vi "Repeat_Meas_if_Unsteady.vi"() -> (5 "Plug in titles":string[](array[string]), 7 "Plug in values":string[](array[string]))   [LabVIEW 2014]
uses:
  Globals/Meas_global.vi
  <vilib>/Analysis/NI_AALPro.lvlib
panel:
  in  "Minumum value to divide by":dbl=100.0 format="%#_13g"
  in  "Acceptable % Drift":dbl=0.5 format="%#_13g"
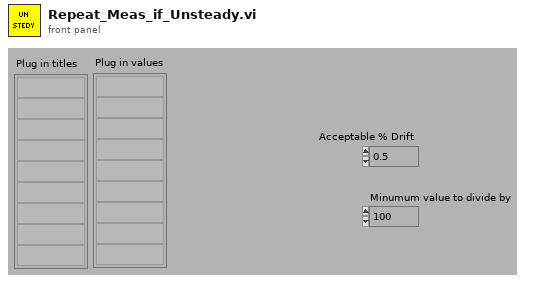
[diagram p1: front panel]
types:
  T1 = typedef "Analysis_info_cluster.ctl" = cluster{"Colour":u32, "Inst type":T2, "Inst name":string, "Symbol":string, "Code name":string, "Extra Info":string, "Inst Array":T3, "Extra Titles":string[], "Extra Values":string[], "U":dbl, "u^2":dbl, "u^3":dbl, "u^4":dbl, "Skew_u":dbl, "Kurt_u":dbl, "Sd Error in Mean":dbl, "% u'/U":dbl, "X":dbl, "Y":dbl, "Z":dbl, "Timescale integral to 25%":dbl, "Sd Error in Variance":dbl, "Calib File":path, "Calib Constants":dbl[], "Output Position":bool, "Full Stats":bool, "Av Sampling Rate":dbl, "Av No of Samples":dbl, "Total Meas Time (s)":dbl, "ADAM Ch Name":string}
  T2 = typedef "Inst_type.ctl" = enum16{"Propeller anemometer", "Raw voltage", "Pressure Transducer", "Pitot-static tube", "Preston tube", "Hot wire", "Cross wire 1", "Cross wire 2", "Generic Linear", "Generic Polynomial", "Generic BackPoly", "Fast FID", "Thermocouple", "Cold wire", "Pulsed Wire", "LDA Vel", "LDA Tran time", "LDA Arr time"}
  T3 = typedef "Instrument_Array.ctl" = enum16{"PWA", "LDA", "Analogue"}
  T4 = typedef "Time_Trace_Cluster.ctl" = cluster{"Weighting":dbl[], "Time (s)":dbl[], "Voltage":dbl[], "Eng Values":dbl[]}
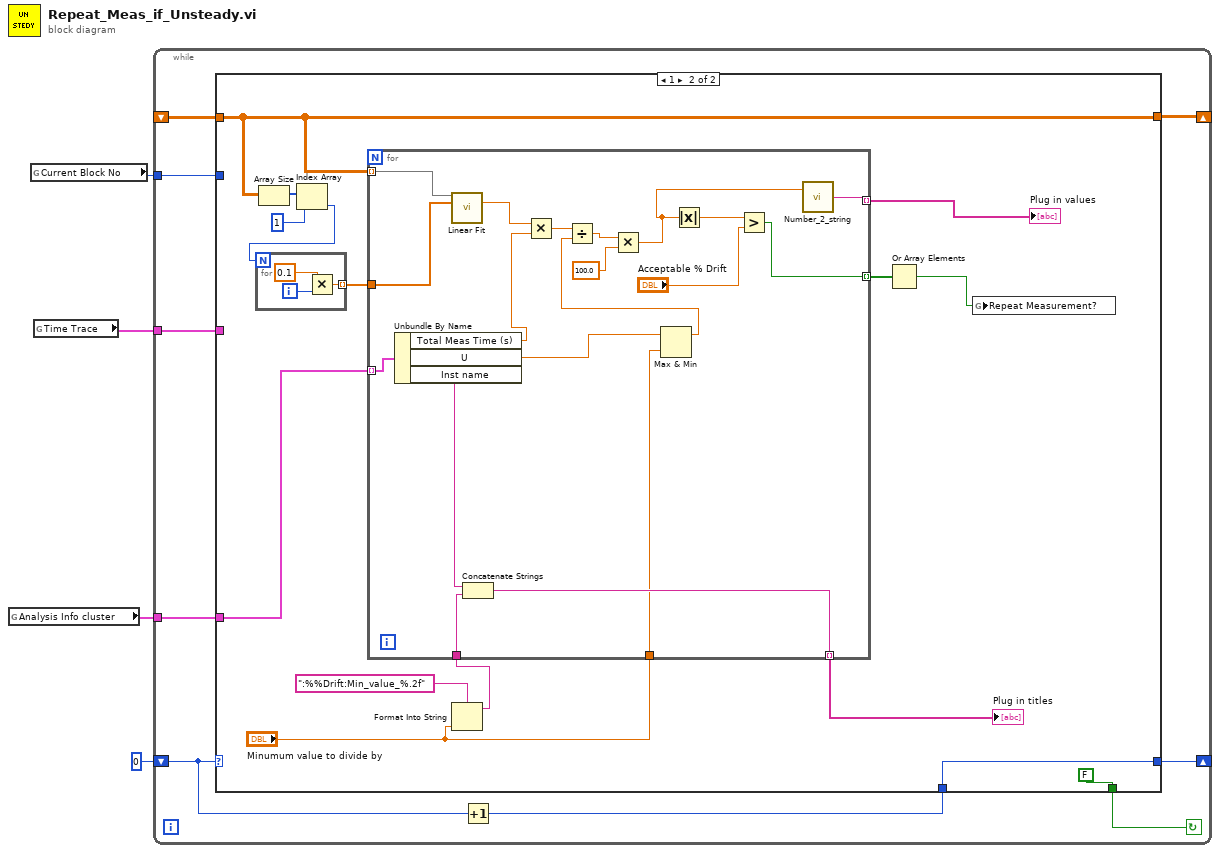
[diagram p0: block diagram]
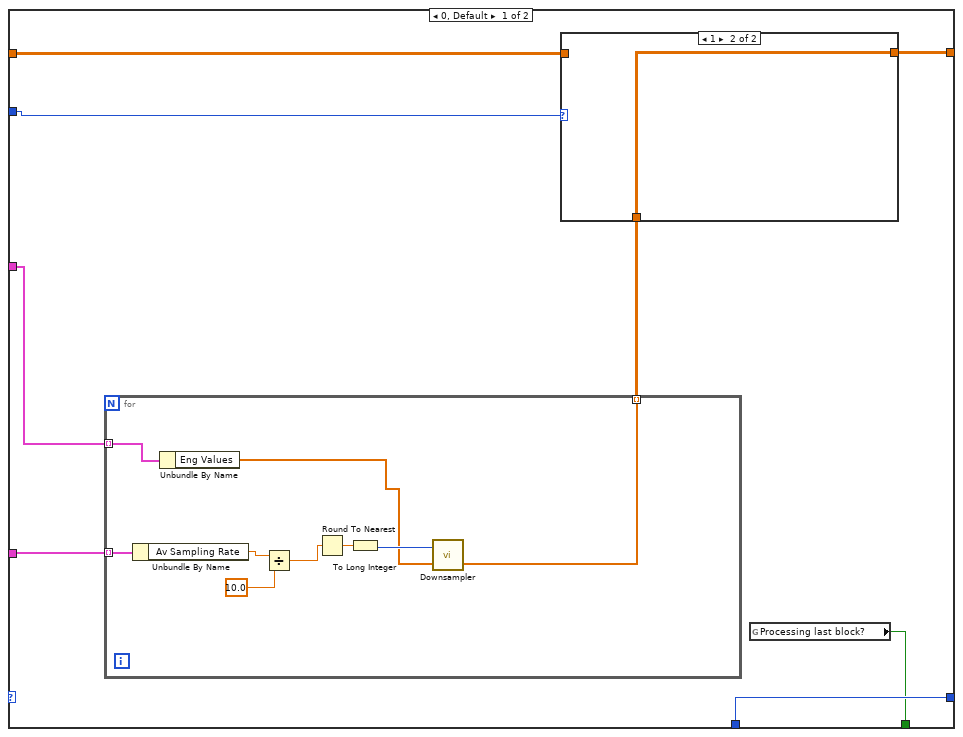
[diagram p2: hidden frame]
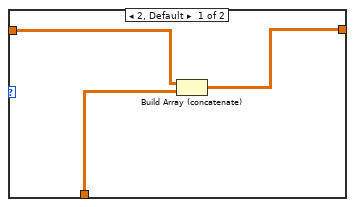
[diagram p3: hidden frame]
diagram:
  n1 = global read "Meas_global.vi" "Analysis Info cluster"() -> (w2:T1[])
  n2 = global read "Meas_global.vi" "Current Block No"() -> (w4:i32)
  n3 = global read "Meas_global.vi" "Time Trace"() -> (w1:T4[])
  n4 = while {
    shift-left: _ -> [w7]
    shift-right: [w8] -> _
    shift-left: 0 -> [w12]
    shift-right: [w10] -> _
    tunnel: w4 -> [w13]
    tunnel: w2 -> [w6]
    tunnel: w1 -> [w5]
    stop <- w9 continue-if-true
    n5 = Increment(x=w12) -> (x+1=w11:i32)
    n6 = case shown="1" w12 {
      tunnel: w13 -> [w20 _]
      tunnel: w11 -> [w21 w48]
      tunnel: [w21 w48] -> w10
      tunnel: [w14 FALSE] -> w9
      tunnel: [w19 w46] -> w8
      tunnel: w7 -> [w18 w46]
      tunnel: w6 -> [w17 w47]
      tunnel: w5 -> [w16 _]
      frame 0, Default {
        n7 = for {
          tunnel: w17 -> [w30] mode=indexing
          tunnel: w16 -> [w29] mode=indexing
          tunnel: [w22] -> w15 mode=indexing
          n8 = Unbundle By Name(w30) -> ("Av Sampling Rate"=w28:dbl)
          n9 = Unbundle By Name(w29) -> ("Eng Values"=w23:dbl[])
          n10 = Divide(x=w28, y=10.0) -> (x/y=w26:dbl)
          n11 = Round To Nearest(number=w26) -> (nearest integer value=w25:dbl)
          n12 = To Long Integer(number=w25) -> (32bit integer=w24:i32)
          n13 = call "Downsampler.vi"("Input Array"=w23, "Averaging samples"=w24) -> ("Downsampled Array"=w22:dbl[])  [unwired: 1 out]
        }
        n14 = case shown="1" w20 {
          tunnel: [w31 w34] -> w19
          tunnel: w18 -> [w33 _]
          tunnel: w15 -> [w32 w34]
          frame 2, Default {
            n15 = Build Array (concatenate)(w33, w32) -> (w31:dbl[][])
          }
          frame 1 {
          }
        }
        n16 = global read "Meas_global.vi" "Processing last block?"() -> (w14:bool)
      }
      frame 1 {
        n17 = Array Size(array=w46) -> (size(s)=w45:i32[])
        n18 = Index Array(array=w45, index=1) -> (element=w43:i32)
        n19 = for {
          N: w43 -> [_]
          tunnel: [w50] -> w42 mode=indexing
          i -> [w52]
          n20 = Multiply(x=0.1, y=w52) -> (x*y=w50:dbl)
        }
        n21 = Format Into String(format string=":%%Drift:Min_value_%.2f", "Minumum value to divide by") -> (resulting string=w35:string)  [unwired: 2 in, 1 out]
        n22 = for {
          tunnel: w47 -> [w71] mode=indexing
          tunnel: [w69] -> w41 mode=indexing
          tunnel: w46 -> [w63] mode=indexing
          tunnel: [w68] -> w40 mode=indexing
          tunnel: w42 -> [w67]
          tunnel: w35 -> [w64]
          tunnel: [w54] -> w39 mode=indexing
          tunnel: "Minumum value to divide by" -> [w53]
          n23 = Unbundle By Name(w71) -> ("Total Meas Time (s)"=w61:dbl, "U"=w66:dbl, "Inst name"=w70:string)
          n24 = call <vilib>:"Linear Fit.vi"("Y"=w63, "X"=w67) -> ("slope"=w62:dbl)  [unwired: 9 in, 4 out]
          n25 = Concatenate Strings(w70, w64) -> (w69:string)
          n26 = Multiply(x=w62, y=w61) -> (x*y=w60:dbl)
          n27 = Max & Min(x=w66, y=w53) -> (max(x,y)=w59:dbl)  [unwired: 1 out]
          n28 = Divide(x=w60, y=w59) -> (x/y=w58:dbl)
          n29 = Multiply(x=w58, y=100.0) -> (x*y=w56:dbl)
          n30 = Absolute Value(x=w56) -> (abs(x)=w65:dbl)
          n31 = Greater?(x=w65, y="Acceptable % Drift") -> (0:w54:bool)
          n32 = call "Number_2_string.vi"("number"=w56) -> ("String"=w68:string)  [unwired: 1 in]
        }
        "Plug in titles" <- w41
        "Plug in values" <- w40
        n33 = Or Array Elements(Boolean array=w39) -> (logical OR=w38:bool)
        n34 = global write "Meas_global.vi" "Repeat Measurement?"(w38) -> ()
      }
    }
  }
